vi "Haversine_distances.vi"(8 "error in":errorcluster caption="entrée d'erreur", 10 "Y":string[][](array[string]), 11 "X":string[][](array[string])) -> (0 "error out":errorcluster caption="sortie d'erreur", 3 "Data":T1)   [LabVIEW 2020]
doc: "Compute the Haversine distance between samples in X and Y\n\nThe Haversine (or great circle) distance is the angular distance between two points on the surface of a sphere. The first distance of each point is assumed to be the latitude, the second is the longitude, given in radians. The dimension of the data must be 2.\n\n\n\nParameters : \n\n- X : array_like, shape (n_samples_1, 2)\n\n- Y: array_like, shape (n_samples_2, 2), optional\n\nReturns : \n\n- distance : {array}, shape (n_samples_1, n_samples_2)"
uses:
  Haversine_distances.lvclass
panel:
  out "Haversine_distances.lvclass":refnum<class "Haversine_distances.lvclass">
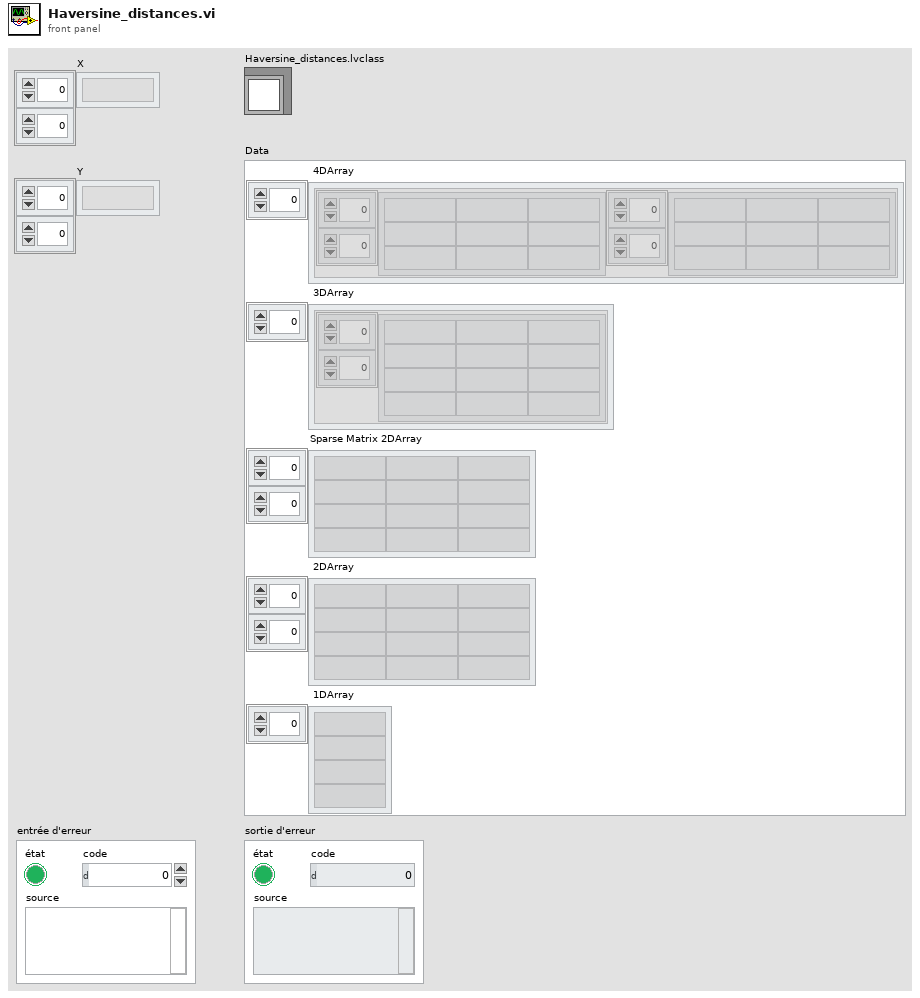
[diagram p1: front panel]
types:
  T1 = cluster{" 4DArray":cluster{"1":string[][], "2":string[][]}[], " 3DArray":cluster{"Tableau":string[][]}[], "Sparse Matrix 2DArray":string[][], " 2DArray":string[][], " 1DArray":string[]}
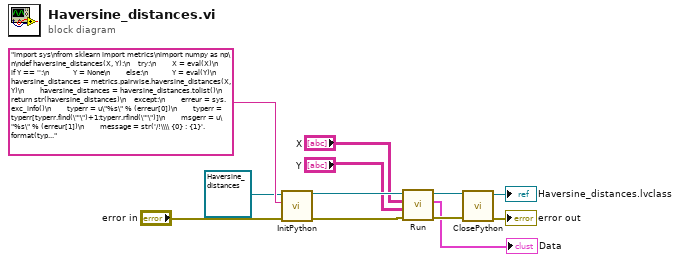
[diagram p0: block diagram]
diagram:
  n1 = call-dynamic "InitPython.vi"("error in (no error)"="error in", "Python Instruction"="import sys\nfrom sklearn import metrics\nimport numpy as np\n\ndef haversine_distances(X, Y):\n    try:\n        X = eval(X)\n        if Y == '':\n            Y = None\n        else:\n            Y = eval(Y)\n        haversine_distances = metrics.pairwise.haversine_distances(X, Y)\n        haversine_distances = haversine_distances.tolist()\n        return str(haversine_distances)\n    except:\n        erreur = sys.exc_info()\n        typerr = u\"%s\" % (erreur[0])\n        typerr = typerr[typerr.find(\"'\")+1:typerr.rfind(\"'\")]\n        msgerr = u\"%s\" % (erreur[1])\n        message = str('/!\\\\ {0} : {1}'. format(typerr,msgerr))\n        return message", "Scikit-learn en entrée"=refnum<class "Haversine_distances.lvclass"> refnum ("Haversine_distances.lvclass")) -> ("error out"=w7:errorcluster, "Scikit-learn en sortie"=w6:refnum<class "Haversine_distances.lvclass">)  [unwired: 7 in]
  n2 = call-dynamic "Run.vi"("error in (no error)"=w7, "Y"="Y", "X"="X", "Haversine_distances.lvclass"=w6) -> ("error out"=w9:errorcluster, "Data"=→"Data":T1, "Haversine_distances.lvclass"=w10:refnum<class "Haversine_distances.lvclass">)  [unwired: 5 in]
  n3 = call-dynamic "ClosePython.vi"("error in (no error)"=w9, "Scikit-learn en entrée"=w10) -> ("error out"=→"error out":errorcluster, "Scikit-learn en sortie"=→"Haversine_distances.lvclass":refnum<class "Haversine_distances.lvclass">)  [unwired: 8 in]
